vi "heinzingerControlMain.vi"(2 "heinzingerControl":T1) -> ()   [LabVIEW 2014]
uses:
  Controls/heinzingerSelect.ctl
  <vilib>/rvi/Emulation/niFpgaGetClockAttributes.vi
  <vilib>/rvi/Emulation/niFpgaSctlEmulationGetInTimedLoop.vi
  <vilib>/rvi/Emulation/niFpgaEmulationReportErrorSimple.vi
  <vilib>/rvi/eio/common/nirviEmuTemplateMethod_errors.vi
  <vilib>/rvi/Emulation/niFpgaCriticalErrorInLSC.vi
  <vilib>/eio/EIONode/EIONode.xnode
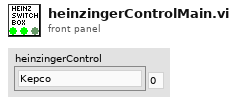
[diagram p1: front panel]
types:
  T1 = typedef "heinzingerSelect.ctl" = enum8{"Kepco", "Heinzinger0", "Heinzinger1", "Heinzinger2"}
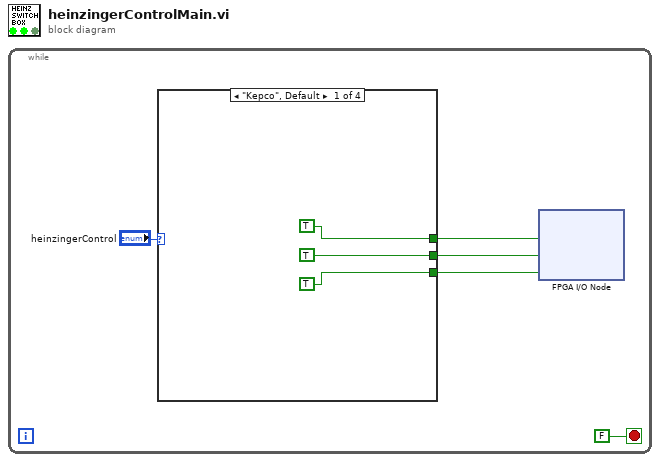
[diagram p0: block diagram]
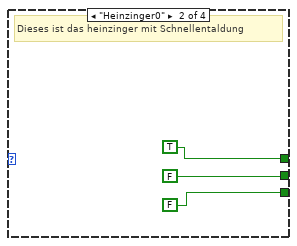
[diagram p2: hidden frame]
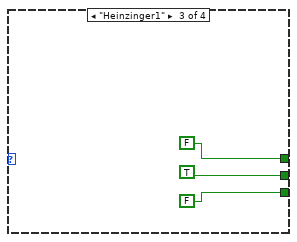
[diagram p3: hidden frame]
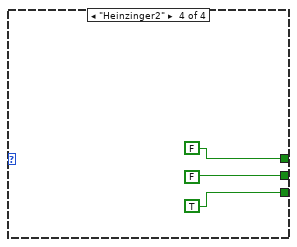
[diagram p4: hidden frame]
diagram:
  n1 = while {
    stop <- FALSE stop-if-true
    n2 = case shown="\"Kepco\", Default" "heinzingerControl" {
      tunnel: [TRUE ("HeinzS0") TRUE ("HeinzS0") FALSE ("HeinzS0") FALSE ("HeinzS0")] -> w4
      tunnel: [TRUE ("HeinzS0") FALSE ("HeinzS0") TRUE ("HeinzS0") FALSE ("HeinzS0")] -> w3
      tunnel: [TRUE ("HeinzS0") FALSE ("HeinzS0") FALSE ("HeinzS0") TRUE ("HeinzS0")] -> w2
      frame "Kepco", Default {
      }
      frame "Heinzinger0" {
        # "Dieses ist das heinzinger mit Schnellentaldung"
      }
      frame "Heinzinger1" {
      }
      frame "Heinzinger2" {
      }
    }
    n3 = xnode "FPGA I/O Node"("HeinzS0"=w4, "HeinzS1"=w3, "HeinzS2"=w2) -> ()  [unwired: 3 in, 3 out]
  }
